vi "Create Scope Info Map.vi"(8 "error in (no error)":errorcluster, 9 "parameters array":T1[](array[typedef]) {"reference position" format="%#_13g"; "min sample rate" format="%#_13p"; "maximum input frequency" format="%#_13p"; "input impedance" items=["1 mega ohm"=0, "50 ohms"=2]; "vertical coupling" items=["AC", "DC", "Ground"]; "probe attenuation" format="%.1f"; "vertical offset" format="%.4f"; "vertical range" format="%#_13g"}, 10 "Pin Names for Scope":string[](array[string]), 11 "connection map":map{string, T4[]}(c390)) -> (0 "error out":errorcluster)   [LabVIEW 2021, in "PMIC Common.lvlib"]
uses:
  PMIC Common.lvlib
  <instrlib>/niScope/Controls/niScope vertical coupling.ctl
  Scope Parameters.ctl
  Instrument Info.ctl
panel:
  out "scope info map":T3(c390)
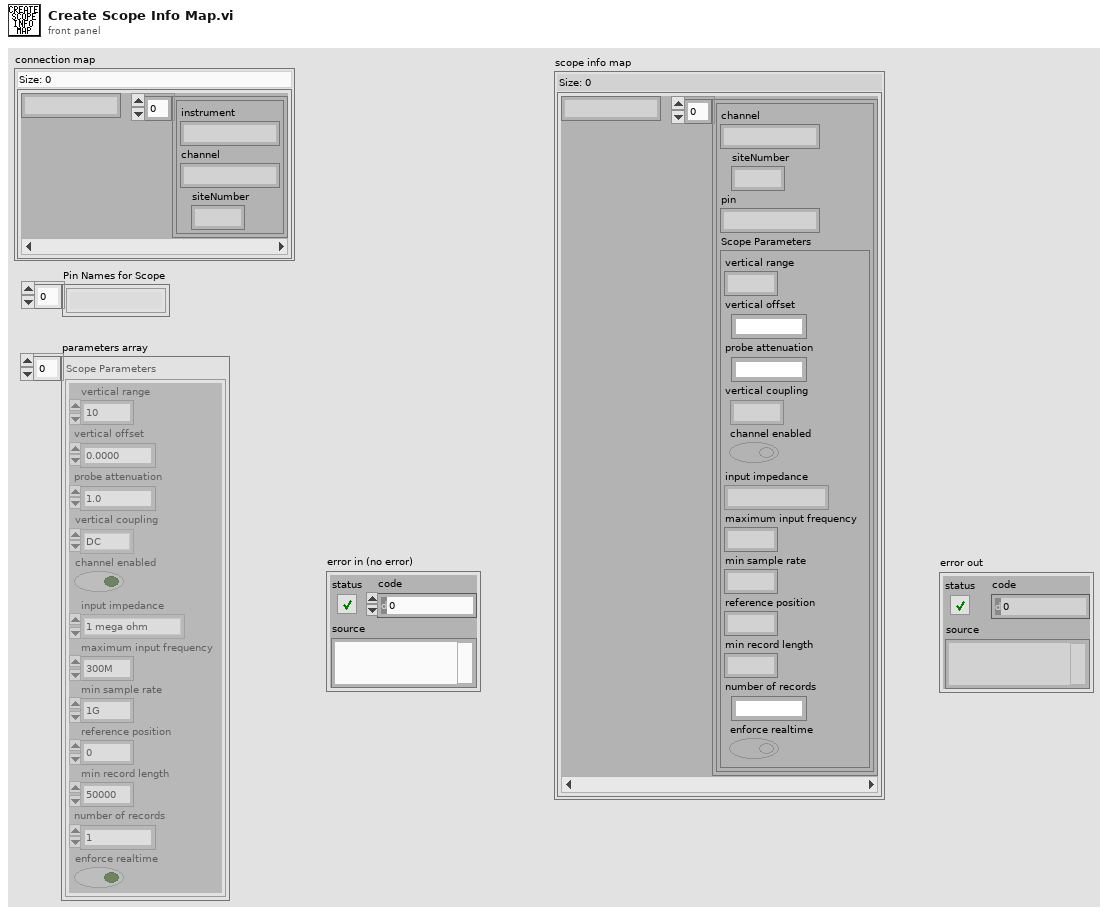
[diagram p1: front panel]
types:
  T1 = typedef "PMIC Common.lvlib/Scope Parameters.ctl" = cluster{"vertical range":dbl, "vertical offset":dbl, "probe attenuation":dbl, "vertical coupling":T2, "channel enabled":bool, "input impedance":u32, "maximum input frequency":dbl, "min sample rate":dbl, "reference position":dbl, "min record length":i32, "number of records":i32, "enforce realtime":bool}
  T2 = typedef "niScope vertical coupling.ctl" = i32
  T3 = map{string, cluster{"channel":string, "siteNumber":i32, "pin":string, "Scope Parameters":T1}[]}
  T4 = typedef "PMIC Common.lvlib/Instrument Info.ctl" = cluster{"instrument":string, "channel":string, "siteNumber":i32}
  T5 = cluster{"channel":string, "siteNumber":i32, "pin":string, "Scope Parameters":T1}[]
  T6 = cluster{"channel":string, "siteNumber":i32, "String":string, "Scope Parameters":T1}
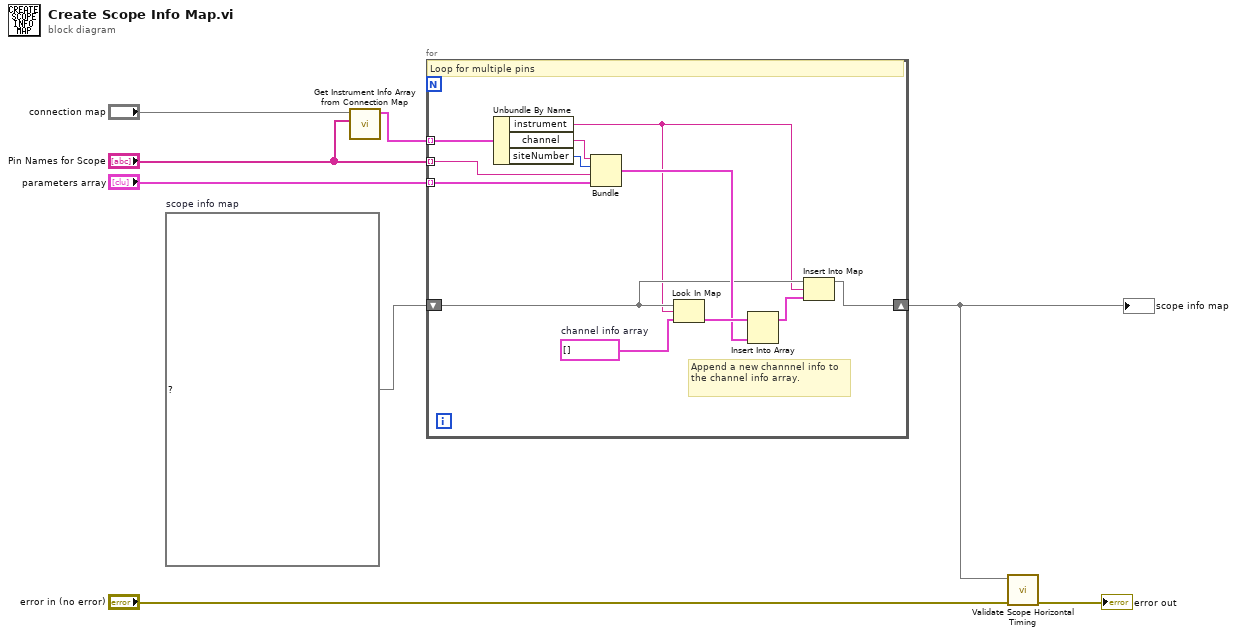
[diagram p0: block diagram]
diagram:
  w7 = T3 {}  # scope info map
  n1 = call "Get Instrument Info Array from Connection Map.vi"("Pin Names for Scope"="Pin Names for Scope", "connection map"="connection map") -> ("instrument info array"=w2:T4[])  [unwired: 9 in]
  n2 = for {
    tunnel: w2 -> [w19] mode=indexing
    tunnel: "parameters array" -> [w10] mode=indexing
    shift-right: [w12] -> w1
    shift-left: w7 -> [w15]
    tunnel: "Pin Names for Scope" -> [w9] mode=indexing
    w11 = T5 []  # channel info array
    # "Append a new channnel info to the channel info array."
    # "Loop for multiple pins"
    n3 = Unbundle By Name(w19) -> ("instrument"=w13:string, "channel"=w20:string, "siteNumber"=w18:i32)
    n4 = Bundle("channel"=w20, "siteNumber"=w18, "String"=w9, "Scope Parameters"=w10) -> (w16:T6)  [unwired: 1 in]
    n5 = Look In Map(map=w15, key=w13, default value=w11) -> (value=w17:T5)  [unwired: 1 out]
    n6 = Insert Into Array(array=w17, new element=w16) -> (w14:T5)  [unwired: 1 in]
    n7 = Insert Into Map(map in=w15, key=w13, value=w14) -> (map out=w12:T3)  [unwired: 2 out]
  }
  "scope info map" <- w1
  n8 = call "Validate Scope Horizontal Timing.vi"("error in (no error)"="error in (no error)", "scope info map"=w1) -> ("error out"=→"error out":errorcluster)  [unwired: 9 in]
